vi "subtract background.vi"(8 "error in (no error)":errorcluster, 11 "Cascade in":refnum<class "Cascade.lvclass">) -> (0 "error out":errorcluster, 3 "Cascade out":refnum<class "Cascade.lvclass">)   [LabVIEW 2012, in "Cascade.lvclass"]
uses:
  Cascade.lvclass
  Cascade.lvclass/Cascade.ctl
  <vilib>/vision/NI_Vision_Development_Module.lvlib
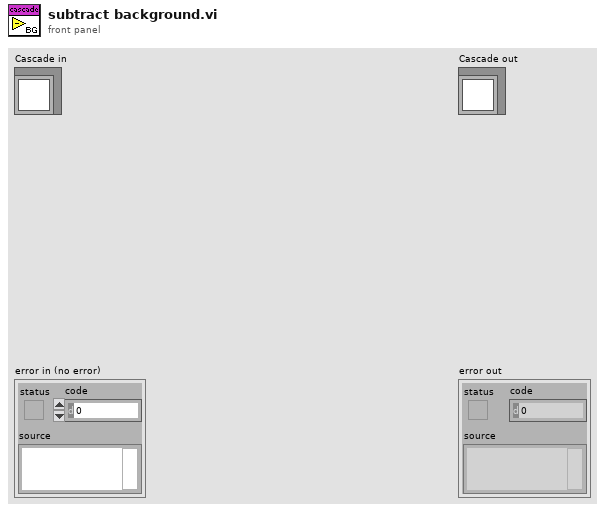
[diagram p1: front panel]
types:
  T1 = typedef "IMAQ Image.ctl" = refnum<image>
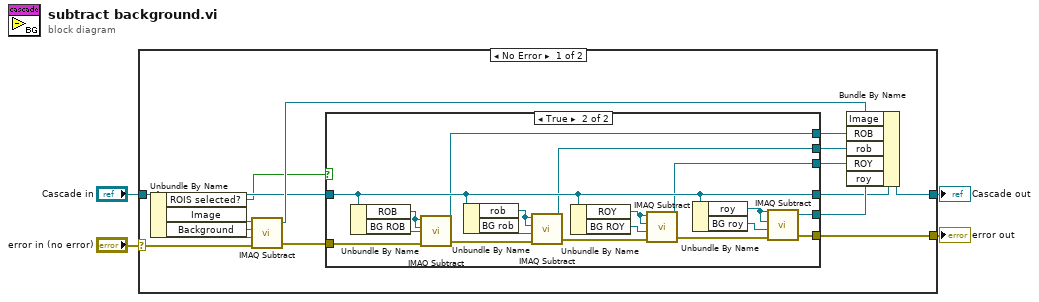
[diagram p0: block diagram]
diagram:
  n1 = case shown="No Error" "error in (no error)" {
    selector: "error in (no error)" -> [w15 w39]
    tunnel: [w7 w39] -> w3
    tunnel: [w13 w38] -> w1
    tunnel: "Cascade in" -> [w6 w38]
    frame No Error {
      n2 = Unbundle By Name(w6) -> ("ROIS selected?"=w5:bool, "Image"=w17:T1, "Background"=w16:T1)
      n3 = call "IMAQ Subtract"("Image Src A"=w17, "Image Dst"=w17, "Image Src B"=w16, "error in (no error)"=w15) -> ("Image Dst Out"=w12:T1, "error out"=w14:errorcluster)  [unwired: 3 in]
      n4 = case shown="True" w5 {
        tunnel: w14 -> [w19 w37]
        tunnel: [_ w34] -> w11
        tunnel: [_ w30] -> w10
        tunnel: [_ w26] -> w9
        tunnel: w6 -> [w18 w20]
        tunnel: [_ w22] -> w8
        tunnel: [w19 w21] -> w7
        tunnel: [w18 w20] -> _
        frame False {
        }
        frame True {
          n5 = Unbundle By Name(w20) -> ("ROB"=w36:T1, "BG ROB"=w35:T1)
          n6 = call "IMAQ Subtract"("Image Src A"=w36, "Image Dst"=w36, "Image Src B"=w35, "error in (no error)"=w37) -> ("Image Dst Out"=w34:T1, "error out"=w33:errorcluster)  [unwired: 3 in]
          n7 = Unbundle By Name(w20) -> ("rob"=w31:T1, "BG rob"=w32:T1)
          n8 = call "IMAQ Subtract"("Image Src A"=w31, "Image Dst"=w31, "Image Src B"=w32, "error in (no error)"=w33) -> ("Image Dst Out"=w30:T1, "error out"=w29:errorcluster)  [unwired: 3 in]
          n9 = Unbundle By Name(w20) -> ("ROY"=w28:T1, "BG ROY"=w27:T1)
          n10 = call "IMAQ Subtract"("Image Src A"=w28, "Image Dst"=w28, "Image Src B"=w27, "error in (no error)"=w29) -> ("Image Dst Out"=w26:T1, "error out"=w25:errorcluster)  [unwired: 3 in]
          n11 = Unbundle By Name(w20) -> ("roy"=w24:T1, "BG roy"=w23:T1)
          n12 = call "IMAQ Subtract"("Image Src A"=w24, "Image Dst"=w24, "Image Src B"=w23, "error in (no error)"=w25) -> ("Image Dst Out"=w22:T1, "error out"=w21:errorcluster)  [unwired: 3 in]
        }
      }
      n13 = Bundle By Name(cluster=w6, "Image"=w12, "ROB"=w11, "rob"=w10, "ROY"=w9, "roy"=w8) -> (w13:refnum<class "Cascade.lvclass">)
    }
    frame Error {
    }
  }
  "error out" <- w3
  "Cascade out" <- w1
